vi "ReloadConfigurationFile.vi"(8 "error in (no error)":errorcluster, 11 "reference In":refnum<class "ModuleAdmin.lvclass">) -> (0 "error out":errorcluster, 3 "reference Out":refnum<class "ModuleAdmin.lvclass">)   [LabVIEW 2018, in "AcPwrPlugins.lvlib"]
doc: "This VI broadcasts a message to Main.vi requesting it to load a new or the same configuration file."
uses:
  AcPwrPlugins.lvlib
  <userlib>/NIST/ModuleAdminLib/ModuleAdmin/ModuleAdmin.lvclass
  AcPwrShared/clEventType.ctl
  AcPwrShared/clDidInit.ctl
  <vilib>/Utility/error.llb/Error Cluster From Error Code.vi
  <vilib>/ErrorRing/Error Ring.xnode
  AcPwrShared/AcPwrShared.lvlib
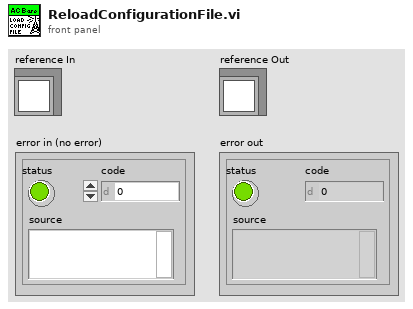
[diagram p1: front panel]
types:
  T1 = typedef "AcPwrShared.lvlib/clBroadcastEvents.ctl" = cluster{"DidInit":refnum<user-event>, "StatusUpdate":refnum<user-event>, "ErrorReport":refnum<user-event>, "DidStop":refnum<user-event>, "PathToINI":refnum<user-event>, "Measurements":refnum<user-event>, "LoadConfigFile":refnum<user-event>, "GetSettings":refnum<user-event>, "SetSettings":refnum<user-event>, "GetType&ID":refnum<user-event>, "GotSettings":refnum<user-event>}
  T2 = typedef "AcPwrShared.lvlib/clDidInit.ctl" = cluster{"Init?":bool, "ModuleAdmin":refnum<class "ModuleAdmin.lvclass">}
  T3 = typedef "AcPwrShared.lvlib/clEventType.ctl" = cluster{"ModuleID":i32, "Data":variant}
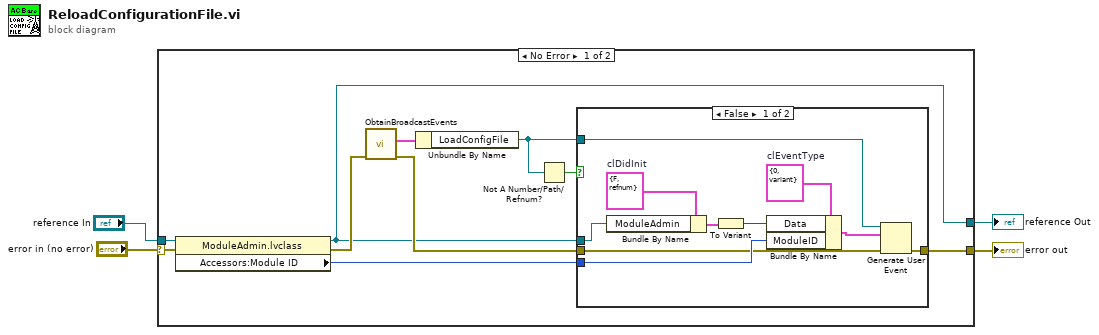
[diagram p0: block diagram]
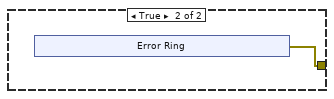
[diagram p2: hidden frame]
diagram:
  n1 = case shown="No Error" "error in (no error)" {
    selector: "error in (no error)" -> [w8 w32]
    tunnel: "reference In" -> [w11 w31]
    tunnel: [w9 w32] -> w3
    tunnel: [w5 w31] -> w1
    frame No Error {
      n2 = property class="ModuleAdmin.lvclass"(reference=w11, error in=w8) -> (reference out=w5:refnum<class "ModuleAdmin.lvclass">, error out=w7:errorcluster, "Accessors:Module ID"=w10:i32)
      n3 = call "ObtainBroadcastEvents.vi"("error in (no error)"=w7) -> ("error out"=w6:errorcluster, "clAcPwrEvents"=w14:T1)  [unwired: 9 in]
      n4 = Unbundle By Name(w14) -> ("LoadConfigFile"=w12:refnum<user-event>)
      n5 = Not A Number/Path/Refnum?(number/path/refnum=w12) -> (NaN/Path/Refnum?=w13:bool)
      n6 = case shown="False" w13 {
        tunnel: w12 -> [w22 _]
        tunnel: [w21 w25] -> w9
        tunnel: w5 -> [w16 _]
        tunnel: w10 -> [w17 _]
        tunnel: w6 -> [w15 _]
        frame False {
          w19 = T2 {"Init?"=FALSE, "ModuleAdmin"=refnum}  # clDidInit
          w24 = T3 {"ModuleID"=0, "Data"=variant}  # clEventType
          n7 = Bundle By Name(cluster=w19, "ModuleAdmin"=w16) -> (w18:T2)
          n8 = To Variant(anything=w18) -> (Variant=w20:variant)
          n9 = Bundle By Name(cluster=w24, "Data"=w20, "ModuleID"=w17) -> (w23:T3)
          n10 = Generate User Event(user event=w22, event data cluster=w23, error in=w15) -> (error out=w21:errorcluster)  [unwired: 1 in, 1 out]
        }
        frame True {
          n11 = xnode "Error Ring"() -> ("error out"=w25:errorcluster)
        }
      }
    }
    frame Error {
    }
  }
  "error out" <- w3
  "reference Out" <- w1
